vi "Update State Data.vi"(8 "error in (no error)":errorcluster, 9 "Data":variant, 10 "Argument":string, 11 "Mouse Action in":refnum<class "Mouse Action.lvclass">) -> (0 "error out":errorcluster, 3 "Mouse Action out":refnum<class "Mouse Action.lvclass">)   [LabVIEW 2020, in "MacroAssert.lvlib" / "Mouse Action.lvclass"]
uses:
  Mouse Action.lvclass
  Mouse Action.lvclass/Mouse Action.ctl
  Action Step/Action Step.lvclass
  CTLs/Mouse Action Type.ctl
  MacroAssert.lvlib
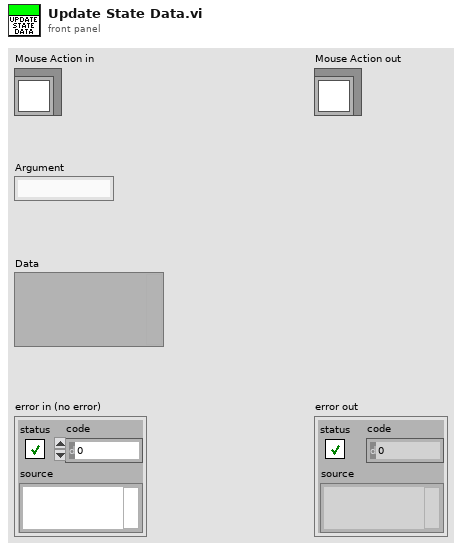
[diagram p1: front panel]
types:
  T1 = typedef "MacroAssert.lvlib/Mouse Action Type.ctl" = enum16{"Click", "Absolute Move", "Absolute Move and Click", "Relative Move", "Relative Move and Click", "Wheel Up", "Wheel Down"}
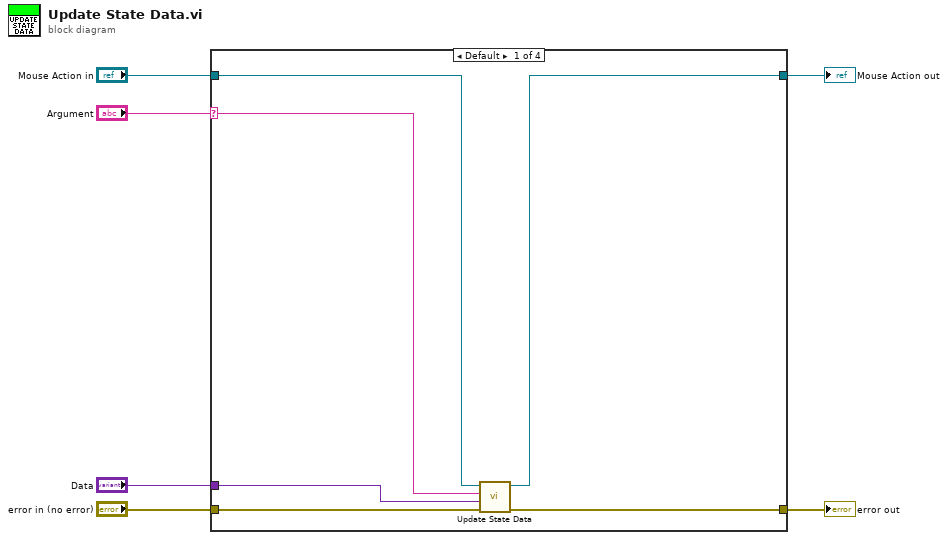
[diagram p0: block diagram]
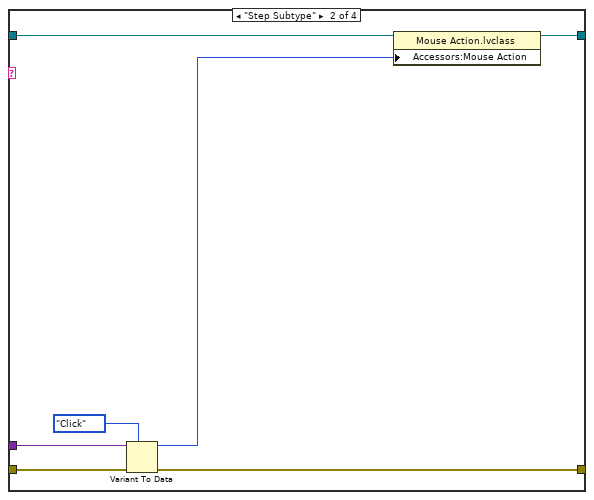
[diagram p2: hidden frame]
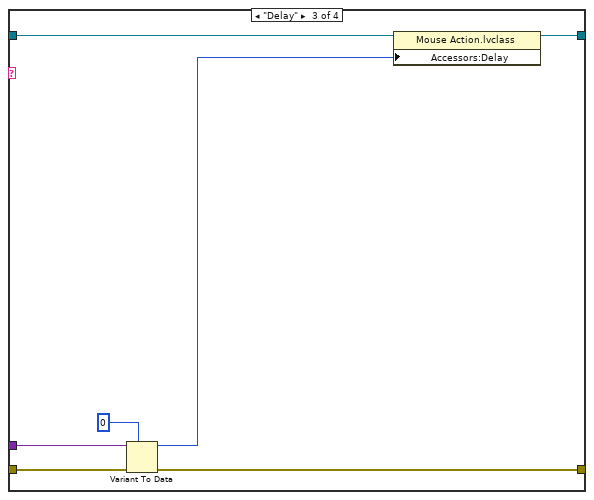
[diagram p3: hidden frame]
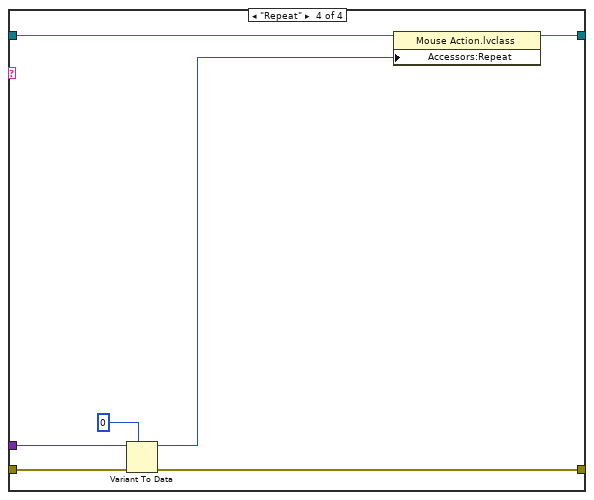
[diagram p4: hidden frame]
diagram:
  n1 = case shown="Default" "Argument" {
    selector: "Argument" -> [w9 _ _ _]
    tunnel: "Mouse Action in" -> [w8 w19 w26 w33]
    tunnel: "error in (no error)" -> [w12 w17 w24 w31]
    tunnel: [w7 w18 w25 w32] -> w2
    tunnel: [w11 w16 w23 w30] -> w1
    tunnel: "Data" -> [w10 w14 w22 w29]
    frame Default {
      n2 = call-parent "Update State Data.vi"("error in (no error)"=w12, "Data"=w10, "Argument"=w9, "Step in"=w8) -> ("error out"=w11:errorcluster, "Step out"=w7:refnum<class "Mouse Action.lvclass">)  [unwired: 6 in]
    }
    frame "Step Subtype" {
      n3 = Variant To Data(error in=w17, type=Mouse_Action_Type."Click" ("Mouse Action Type"), Variant=w14) -> (data=w13:T1, error out=w16:errorcluster)
      n4 = property class="Mouse Action.lvclass"(reference=w19, "Accessors:Mouse Action"=w13) -> (reference out=w18:refnum<class "Mouse Action.lvclass">)  [unwired: 1 in, 1 out]
    }
    frame "Delay" {
      n5 = Variant To Data(error in=w24, type=0, Variant=w22) -> (data=w21:i32, error out=w23:errorcluster)
      n6 = property class="Mouse Action.lvclass"(reference=w26, "Accessors:Delay"=w21) -> (reference out=w25:refnum<class "Mouse Action.lvclass">)  [unwired: 1 in, 1 out]
    }
    frame "Repeat" {
      n7 = Variant To Data(error in=w31, type=0, Variant=w29) -> (data=w28:i32, error out=w30:errorcluster)
      n8 = property class="Mouse Action.lvclass"(reference=w33, "Accessors:Repeat"=w28) -> (reference out=w32:refnum<class "Mouse Action.lvclass">)  [unwired: 1 in, 1 out]
    }
  }
  "error out" <- w1
  "Mouse Action out" <- w2
